vi "3.7-UDP Debug Indicator.vi"() -> (0 "4.7-UDP Debug":T2)   [LabVIEW 2010]
uses:
  4-High Neurons/4.0-Timing Badass.ctl
  3.0-Global.vi
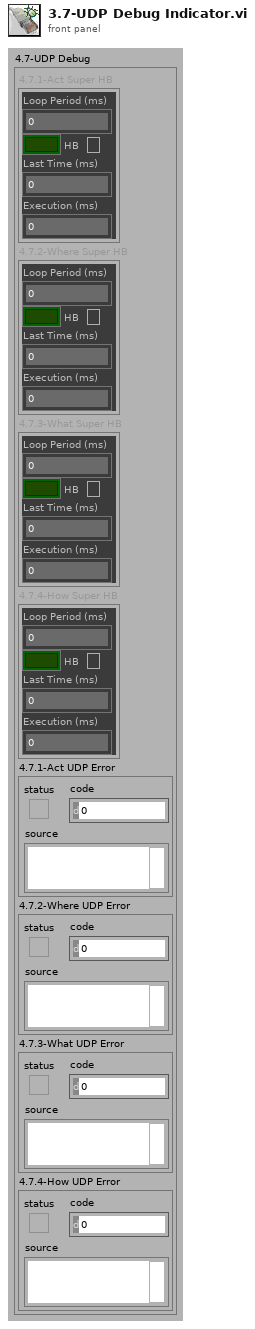
[diagram p1: front panel]
types:
  T1 = typedef "4.0-Timing Badass.ctl" = cluster{"Loop Period (ms)":u32, "HB":bool, "Last Time (ms)":u32, "Execution (ms)":u32}
  T2 = cluster{"4.7.1-Act Super HB":T1, "4.7.2-Where Super HB":T1, "4.7.3-What Super HB":T1, "4.7.4-How Super HB":T1, "4.7.1-Act UDP Error":errorcluster, "4.7.2-Where UDP Error":errorcluster, "4.7.3-What UDP Error":errorcluster, "4.7.4-How UDP Error":errorcluster}
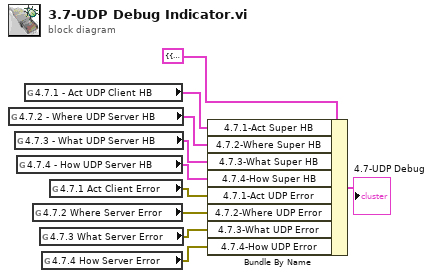
[diagram p0: block diagram]
diagram:
  n1 = global read "3.0-Global.vi" "4.7.2 - Where UDP Server HB"() -> (w3:T1)
  n2 = global read "3.0-Global.vi" "4.7.3 - What UDP Server HB"() -> (w2:T1)
  n3 = global read "3.0-Global.vi" "4.7.4 - How UDP Server HB"() -> (w1:T1)
  n4 = global read "3.0-Global.vi" "4.7.1 - Act UDP Client HB"() -> (w4:T1)
  n5 = global read "3.0-Global.vi" "4.7.2 Where Server Error"() -> (w6:errorcluster)
  n6 = global read "3.0-Global.vi" "4.7.3 What Server Error"() -> (w7:errorcluster)
  n7 = global read "3.0-Global.vi" "4.7.4 How Server Error"() -> (w8:errorcluster)
  n8 = global read "3.0-Global.vi" "4.7.1 Act Client Error"() -> (w5:errorcluster)
  n9 = Bundle By Name(cluster=T2 {"4.7.1-Act Super HB"={"Loop Period (ms)"=0, "HB"=FALSE, "Last Time (ms)"=0, "Execution (ms)"=0}, "4.7.2-Where Super HB"={"Loop Period (ms)"=0, "HB"=FALSE, "Last Time (ms)"=0, "Execution (ms)"=0}, "4.7.3-What Super HB"={"Loop Period (ms)"=0, "HB"=FALSE, "Last Time (ms)"=0, "Execution (ms)"=0}, "4.7.4-How Super HB"={"Loop Period (ms)"=0, "HB"=FALSE, "Last Time (ms)"=0, "Execution (ms)"=0}, "4.7.1-Act UDP Error"={"status"=FALSE, "code"=0, "source"=""}, "4.7.2-Where UDP Error"={"status"=FALSE, "code"=0, "source"=""}, "4.7.3-What UDP Error"={"status"=FALSE, "code"=0, "source"=""}, "4.7.4-How UDP Error"={"status"=FALSE, "code"=0, "source"=""}} ("4.7-UDP Debug"), "4.7.1-Act Super HB"=w4, "4.7.2-Where Super HB"=w3, "4.7.3-What Super HB"=w2, "4.7.4-How Super HB"=w1, "4.7.1-Act UDP Error"=w5, "4.7.2-Where UDP Error"=w6, "4.7.3-What UDP Error"=w7, "4.7.4-How UDP Error"=w8) -> (→"4.7-UDP Debug":T2)
